vi "io_set_VISA_timeout.vi"(8 "error in":errorcluster, 10 "VISA Timeout":u32=5000, 11 "VISA resource name":refnum<visa-resource-name>) -> (0 "error out":errorcluster, 2 "Old VISA Timeout":u32, 3 "VISA resource name out":refnum<visa-resource-name>)   [LabVIEW 2014, in "rszvl_rsidr_core.lvlib"]
uses:
  rszvl_rsidr_core.lvlib
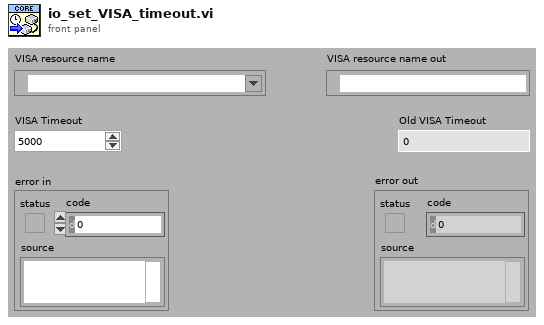
[diagram p1: front panel]
types:
  T1 = typedef "rszvl_rsidr_core.lvlib/type_Session_Data.ctl" = cluster{"Instr type":string, "Instr type for err. msg.":string, "Installed Options":string[], "OPC Timeout":i32, "Query Instrument Status":bool, "Check Range":bool, "Check Options":bool, "Add LF to Write":bool, "Simulate":bool, "Logging":bool, "Logging params":variant, "Interface Type":enum16{"Unknown", "GPIB", "VXI", "GPIB_VXI", "ASRL", "PXI", "TCPIP", "USB", "SOCKET"}, "Fast Sweep":i32, "AdditionalFlags":i32, "WaitBeforeWrite":i32, "WaitBeforeRead":i32, "BinDataChunkSize":i64}
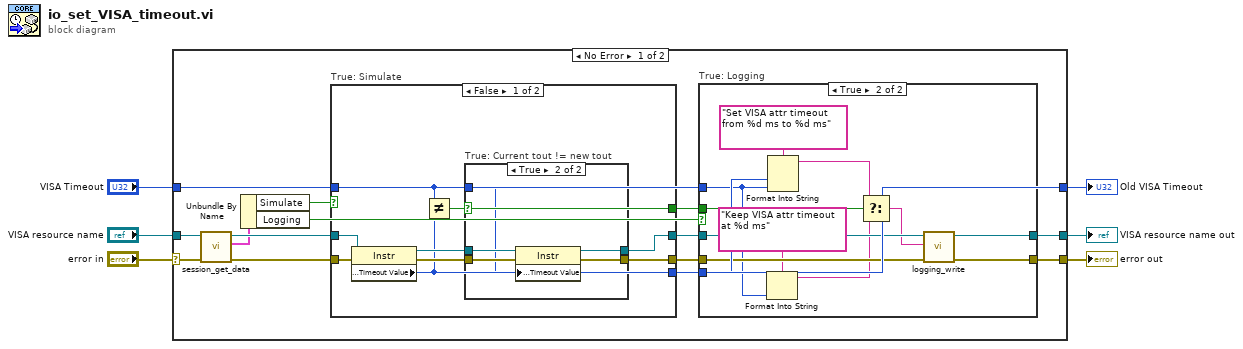
[diagram p0: block diagram]
diagram:
  n1 = case shown="No Error" "error in" {
    selector: "error in" -> [w20 w55]
    tunnel: [w11 w55] -> w4
    tunnel: "VISA resource name" -> [w19 w54]
    tunnel: [w8 w54] -> w3
    tunnel: [w10 w56] -> w2
    tunnel: "VISA Timeout" -> [w14 w56]
    frame No Error {
      n2 = call "session_get_data.vi"("error in"=w20, "VISA resource name"=w19) -> ("error out"=w9:errorcluster, "Session User Data out"=w17:T1, "VISA resource name out"=w18:refnum<visa-resource-name>)  [unwired: 7 in]
      n3 = Unbundle By Name(w17) -> ("Simulate"=w16:bool, "Logging"=w15:bool)
      n4 = case "True: Simulate" shown="False" w16 {
        tunnel: w9 -> [w43 w53]
        tunnel: [w41 w53] -> w12
        tunnel: [w40 w52] -> w13
        tunnel: w18 -> [w39 w52]
        tunnel: [w37 w51] -> w10
        tunnel: w14 -> [w36 w51]
        tunnel: [w35 _] -> w7
        frame False {
          n5 = property on="Property Node" class="Instr"(reference=w39, error in=w43) -> (reference out=w38:refnum<visa-resource-name>, error out=w42:errorcluster, "General Settings:Timeout Value"=w37:u32)
          n6 = Not Equal?(x=w36, y=w37) -> (x != y?=w35:bool)
          n7 = case "True: Current tout != new tout" shown="True" w35 {
            tunnel: w42 -> [w44 w50]
            tunnel: [w44 w49] -> w41
            tunnel: [w45 w48] -> w40
            tunnel: w38 -> [w45 w47]
            tunnel: w36 -> [_ w46]
            frame False {
            }
            frame True {
              n8 = property on="Property Node" class="Instr"(reference=w47, error in=w50, "General Settings:Timeout Value"=w46) -> (reference out=w48:refnum<visa-resource-name>, error out=w49:errorcluster)
            }
          }
        }
        frame True {
        }
      }
      n9 = case "True: Logging" shown="True" w15 {
        tunnel: w14 -> [_ w28]
        tunnel: w13 -> [w21 w34]
        tunnel: w12 -> [w22 w31]
        tunnel: [w22 w30] -> w11
        tunnel: w10 -> [_ w32]
        tunnel: [w21 w29] -> w8
        tunnel: w7 -> [_ w26]
        frame False {
        }
        frame True {
          n10 = Format Into String(format string="Keep VISA attr timeout at %d ms", w28) -> (resulting string=w24:string)  [unwired: 2 in, 1 out]
          n11 = Format Into String(format string="Set VISA attr timeout from %d ms to %d ms", w32, w28) -> (resulting string=w25:string)  [unwired: 2 in, 1 out]
          n12 = Select(t=w25, s=w26, f=w24) -> (s? t:f=w23:string)
          n13 = call "logging_write.vi"("error in"=w31, "String to write"=w23, "VISA resource name"=w34) -> ("error out"=w30:errorcluster, "VISA resource name out"=w29:refnum<visa-resource-name>)  [unwired: 7 in]
        }
      }
    }
    frame Error {
    }
  }
  "VISA resource name out" <- w3
  "error out" <- w4
  "Old VISA Timeout" <- w2
